vi "subVI1.vi"(10 "Boolean":bool, 11 "Fahrenheit":dbl) -> (3 "Celsius":dbl)   [LabVIEW 2017]
doc: "This VI will recieve a temperature in Farenheit and will return a temperature in celsius"
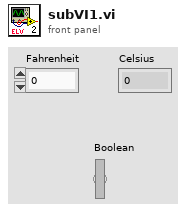
[diagram p1: front panel]
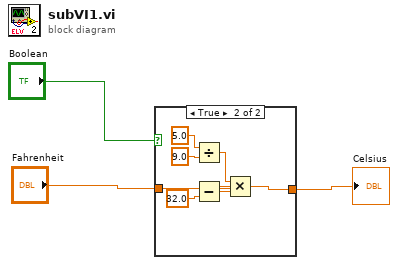
[diagram p0: block diagram]
diagram:
  n1 = case shown="True" "Boolean" {
    tunnel: [w4 w10] -> w3
    tunnel: "Fahrenheit" -> [w4 w5]
    frame False {
    }
    frame True {
      n2 = Divide(x=5.0, y=9.0) -> (x/y=w7:dbl)
      n3 = Subtract(x=w5, y=32.0) -> (x-y=w6:dbl)
      n4 = Multiply(x=w7, y=w6) -> (x*y=w10:dbl)
    }
  }
  "Celsius" <- w3
